vi "dataAcq_get_interferogram.vi"(0 "reference":refnum<class "OSA300.lvclass">, 5 "error in (no error)":errorcluster) -> (14 "duplicate reference":refnum<class "OSA300.lvclass">, 19 "error out":errorcluster)   [LabVIEW 2010, in "OSA300.lvclass"]
doc: "Reads data from spectrometer and updates labview buffer interferogram Y array, X is equidistant, (x min and max). See buffer_get.vi for labview buffer data access. \n\nX: optical path length\nY: ADC value"
uses:
  OSA300.lvclass
  OSA.lvclass
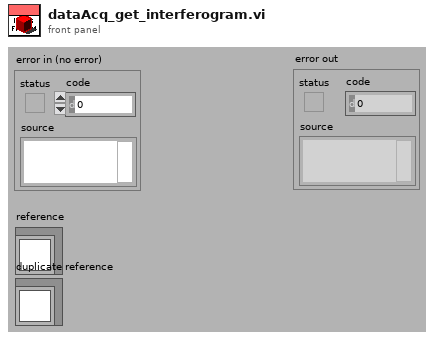
[diagram p1: front panel]
types:
  T1 = cluster{"index tot":i32, "waveMin (cm-1)":i32, "waveMax (cm-1)":i32, "gain":i32, "offset":i32, "index DUT":i32}[]
  T2 = cluster{"index tot":i32, "waveMin (cm-1)":i32, "waveMax (cm-1)":i32, "gain":i32, "offset":i32, "index DUT":i32}
  T3 = typedef "OSA20X.lvclass/ObjectAttributes.ctl" = cluster{"Stop":bool, "dataType":T4, "spectrometerIdx":u16, "buffer size interferogram":i32, "interferogram":cluster{"new":bool, "plot_x_ min":sgl, "plot_x_max":sgl, "plot_y_min":sgl, "plot_y_max":sgl, "Graph Intrfrgrm":T5, "timeStamp":u32, "signal (%)":dbl, "traces":cluster{"idx":u32, "broadBand":bool, "monoChromatic":bool, "peakToPeakSignal":dbl, "peakToPeakPos":dbl}[], "traces idx last":i32}, "spectrum":cluster{"new":bool, "plot_x_min":sgl, "plot_x_max":sgl, "plot_unit_x":T6, "plot_unit_y":T7, "plot_y_min":sgl, "plot_y_max":sgl, "Graph Spectrum":T5, "timeStamp":u32, "X_VAL_OPTIONS":enum16{"MIN_MAX", "ARRAY"}, "traces":cluster{"idx":u32}[], "traces idx last":i32}, "Thorlabs_OSA_64.lvclass:queue_action.ctlqueue ref":refnum<queue>, "action":T8, "plot zoom step":dbl, "buffer semaphore":T9, "acq stopped":bool, "dataType active":T4, "temperature (degr C)":sgl, "pressure (hPa)":sgl, "rel humidity (%)":sgl, "settings":cluster{"resolution":T10, "sensitivity":T11, "Average":bool, "average nr":u32, "apodisation":T12, "acq delay (ms)":u32, "airMesure":T13, "wmtr on":bool, "intfgrm_smooth_width":u16, "intfgrm_smooth_nrOfPasses":u16, "intfgrm_smooth":T14, "phaseCorrection":T15, "zeroFill":u8, "spectr_smooth":T14, "spectr_smooth_width":u16, "spectr_smooth_nrOfPasses":u16, "resolution (/cm)":sgl, "REF wavelength, (nm)":dbl, "gain_idx":u16, "gainAuto":bool, "gain_relative":dbl, "PD sensitivity mode":T16, "PD senseMode implemented":bool, "SensorTemperature implemented":bool, "SensorPressure implemented":bool, "SensorHumidity implemented":bool}, "peaks position":sgl[], "peaks width":sgl[], "peaks height":sgl[], "peaks max nr":u32, "peaks latest nr":i32, "peaks new":bool, "power":dbl, "power new":bool, "path":string, "wavelength (WNr)":dbl, "wavelength new":bool, "buffer size spectrum":i32, "status":string, "VI reference":refnum<vi>, "funcPointer":u64, "libraryPointer":u64, "singleAcquisition":bool, "coherenceLength (cm)":dbl, "coherenceLength new":bool, "spectrometer model":string, "spectrometer serial nr":string, "peaks thld left":sgl[], "peaks thld right":sgl[], "coherenceLength error (cm)":dbl, "ADC bits":u16, "peaks position centroid":sgl[], "peaks height centroid":sgl[], "OSA series":T17, "channel":u16, "channels_nr":i32, "channel stiched":u32}
  T4 = typedef "OSA20X.lvclass/acq_dataType.ctl" = enum16{"none", "interferogram", "spectrum"}
  T5 = typedef "OSA20X.lvclass/graph_intensity.ctl" = refnum<vi>
  T6 = typedef "OSA20X.lvclass/spectrum_x_unit.ctl" = enum16{"wavenr/cm", "THz", "eV", "nm_air", "nm_vac"}
  T7 = typedef "OSA20X.lvclass/y_unit.ctl" = enum16{"ADC counts", "dBm pwr absolute", "dBm pwr density", "mW pwr absolute", "mW pwr density"}
  T8 = typedef "OSA20X.lvclass/queue_action.ctl" = enum16{"none", "stop", "GUI_plotInterferogram", "GUI_plotSpectrum", "GUI_plotInterferogramRescale", "GUI_plotSpectrumRescale", "GUI_plotInterferogramReset", "GUI_plotSpectrumReset", "GUI_plotInterferogramAutoScaleY", "GUI_plotSpectrumAutoScaleY", "GUI_plotInterferogramZoomOut", "GUI_plotSpectrumZoomOut", "GUI_plotInterferogramPane", "GUI_plotSpectrumPane", "GUI_plotInterferogramZoomMouse", "GUI_plotSpectrumZoomMouse", "ENVIRONMENT temperature", "ENVIRONMENT pressure", "MODE_resolution set", "MODE_resolution get", "MODE_sensitivity set", "MODE_sensitivity get", "MODE_PDTemperature set", "MODE_PDTemperature get", "REBOOT/RESET firmware", "ACQASYNC_acquireSingleSpectrum", "ACQASYNC_continuous start", "ACQASYNC_continuous stop\n", "ACQASYNC_get last interferogram", "ACQASYNC_get last spectrum", "ACQASYNC_get last waveNr", "ACQOPT_interferogram smoothing set", "ACQOPT_interferogram smoothing get", "ACQOPT_spectrum smoothing set", "ACQOPT_spectrum smoothing get", "ACQOPT_apodisation type set", "ACQOPT_apodisation type get", "ACQOPT_phase correction type set", "ACQOPT_phase correction type get", "ACQOPT_acqIntervall_set", "ACQOPT_acqIntervall_get", "ACQOPT_average spectrum set", "ACQOPT_average spectrum get", "ACQOPT_rolling average set", "ACQOPT_rolling average get", "ACQOPT_zero fill factor set", "ACQOPT_zero fill factor get", "ACQOPT_cycle counting set", "ACQOPT_cycle counting get", "ACQOPT_air measure option set", "ACQOPT_air measure option get", "ACQOPT_gainLevel auto get", "ACQOPT_gainLevel auto set", "ACQOPT_gainLevel get", "ACQOPT_gainLevel set", "ACQOPT_getAll", "INSTRUMENT_PROPERTY_range_WaveNr_min", "INSTRUMENT_PROPERTY_range_WaveNr_max", "INSTRUMENT_PROPERTY_reference_wavelength_cm^-1", "INSTRUMENT_PROPERTY_samplesPerRefPeriod", "INSTRUMENT_PROPERTY_resolution_waveNrPercm", "INSTRUMENT_PROPERTY_availableGainLevels", "INSTRUMENT_PROPERTY_status", "CONVERT", "ANALYSE_POWER", "ANALYSE_PEAKS", "ANALYSE_WAVELENGTH", "ANALYSE_SPECTRUM", "ANALYSE_INTERFEROGRAM", "ANALYSE_COHERENCE_LENGTH", "MATH", "MATH_power", "MATH_peaks", "FILE", "miscellaneous"}
  T9 = typedef "Semaphore RefNum" = refnum<k1>
  T10 = typedef "OSA20X.lvclass/resolution.ctl" = enum16{"low", "high"}
  T11 = typedef "OSA20X.lvclass/sensitivityMode.ctl" = enum16{"low", "low medium", "high medium", "high"}
  T12 = typedef "OSA20X.lvclass/apodisation.ctl" = enum16{"NONE", "NORTON_BEER_WEAK", "NORTON_BEER_MEDIUM", "NORTON_BEER_STRONG", "TRIANGULAR", "COSINE", "HANN", "HAMMING", "BLACKMANHARRIS3", "BLACKMANHARRIS4", "GAUSSIAN"}
  T13 = typedef "OSA20X.lvclass/airMeasure.ctl" = enum16{"TEMPERATURE", "PRESSURE"}
  T14 = typedef "OSA20X.lvclass/smoothing.ctl" = enum16{"NONE", "BINOMIAL", "SAVITSKY_GOLAY", "FOURIER", "MOVING_AVERAGE", "GAUSSIAN"}
  T15 = typedef "OSA20X.lvclass/phaseCorrection.ctl" = enum16{"NONE", "MERTZ", "FORMAN", "MERTZ_FILE", "FORMAN_FILE", "FUTURE COMP."}
  T16 = typedef "OSA20X.lvclass/PDTemperatureMode.ctl" = enum16{"cool: better sensitivity/noise floor", "warm: extended wl range"}
  T17 = typedef "OSA_series.ctl" = enum16{"OSA200", "OSA300", "UNKNOWN"}
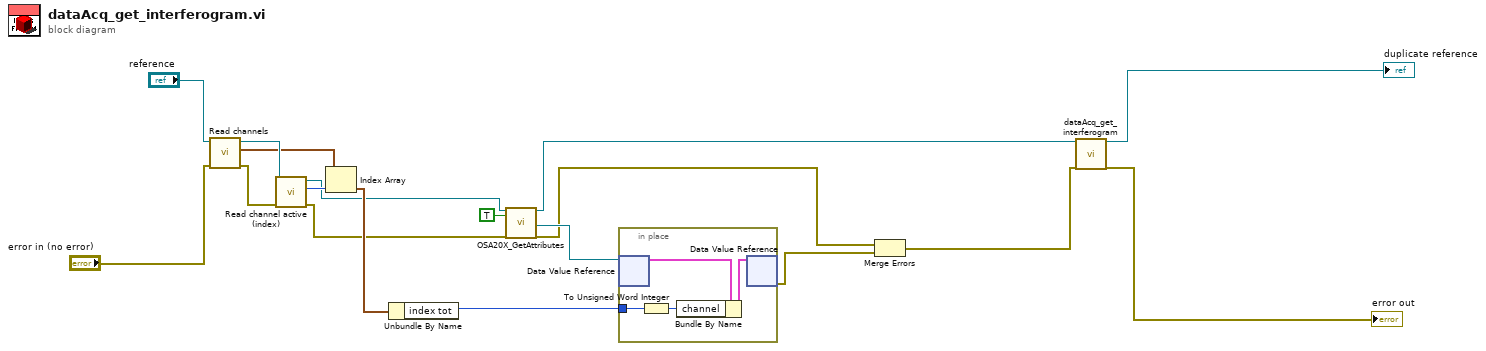
[diagram p0: block diagram]
diagram:
  n1 = call "Read channels.vi"("error in (no error)"="error in (no error)", "OSA300 in"="reference") -> ("error out"=w14:errorcluster, "channels"=w12:T1, "OSA300 out"=w13:refnum<class "OSA300.lvclass">)  [unwired: 7 in]
  n2 = call "Read channel active (index).vi"("error in (no error)"=w14, "OSA300 in"=w13) -> ("error out"=w4:errorcluster, "channel active (index)"=w11:i32, "OSA300 out"=w7:refnum<class "OSA300.lvclass">)  [unwired: 7 in]
  n3 = Index Array(array=w12, index=w11) -> (element=w10:T2)
  n4 = Unbundle By Name(w10) -> ("index tot"=w5:i32)
  n5 = call "OSA20X_GetAttributes.vi"("reference in"=w7, "OnlyGetDvrReference(False)"=TRUE, "error in (no error)"=w4) -> ("reference out"=w6:refnum<class "OSA300.lvclass">, "DataRef"=w8:refnum<data-value>, "error out"=w3:errorcluster)  [unwired: 13 in, 1 out]
  n6 = in-place {
    in-place-border: w5 -> [w20]
    n7 = in-place-dvr #1(w8) -> (w21:T3)  [unwired: 1 out]
    n8 = To Unsigned Word Integer(number=w20) -> (unsigned 16bit integer=w19:u16)
    n9 = Bundle By Name(cluster=w21, "channel"=w19) -> (w22:T3)
    n10 = in-place-dvr #1(w22) -> (w2:errorcluster)  [unwired: 1 out]
  }
  n11 = Merge Errors(w3, w2) -> (w1:errorcluster)
  n12 = call-parent "dataAcq_get_interferogram.vi"("reference"=w6, "error in (no error)"=w1) -> ("duplicate reference"=→"duplicate reference":refnum<class "OSA300.lvclass">, "error out"=→"error out":errorcluster)  [unwired: 16 in]
